vi "PickAndPlaceOnTape.vi"() -> ()   [LabVIEW 2021]
panel:
  in  "GoHome":bool
  in  "Operations":T1={"GoToToolPos"=TRUE, "PickTool"=TRUE, "GoToSenPCB"=TRUE, "PickSiPCB"=TRUE, "GoToBP"=TRUE, "DropTool"=TRUE}
  out "ZoneBasedFileNameStarting":string
  in  "Tape_PositionPartialFileName":string="Other_Position.txt"
  in  "PUT_PositionPartialFileName":string="PUT_Position.txt"
  in  "AssemblyPositionPartialFileName":string="Other_Position.txt"
  in  "BaseDirectory":string="C:\\Users\\TTUHEP\\Documents\\LabVIEW\\GantryPrograms\\Configs\\"
  out "Assembly_XYZU":dbl[](array[numeric])
  out "PUT_XYZU":dbl[](array[numeric])
  out "PUT rotation":dbl
  in  "FastZDrop":dbl=65.0
  in  "FastZToolPick":dbl=85.0
  in  "FastZSiPCBPick":dbl=65.0
  in  "LineNo":u8
  in  "ZSpeed":dbl=10.0
  in  "XYSpeed":dbl=100.0
  out "BPHBXYZU":dbl[](array[numeric])
  out "Error Out":errorcluster
  in  "Error In":errorcluster
  in  "VacuumStates":path=path "C:/Users/TTUHEP/Documents/LabVIEW/GantryPrograms/Configs/TapeCompPickPlaceVacuumStates.json"
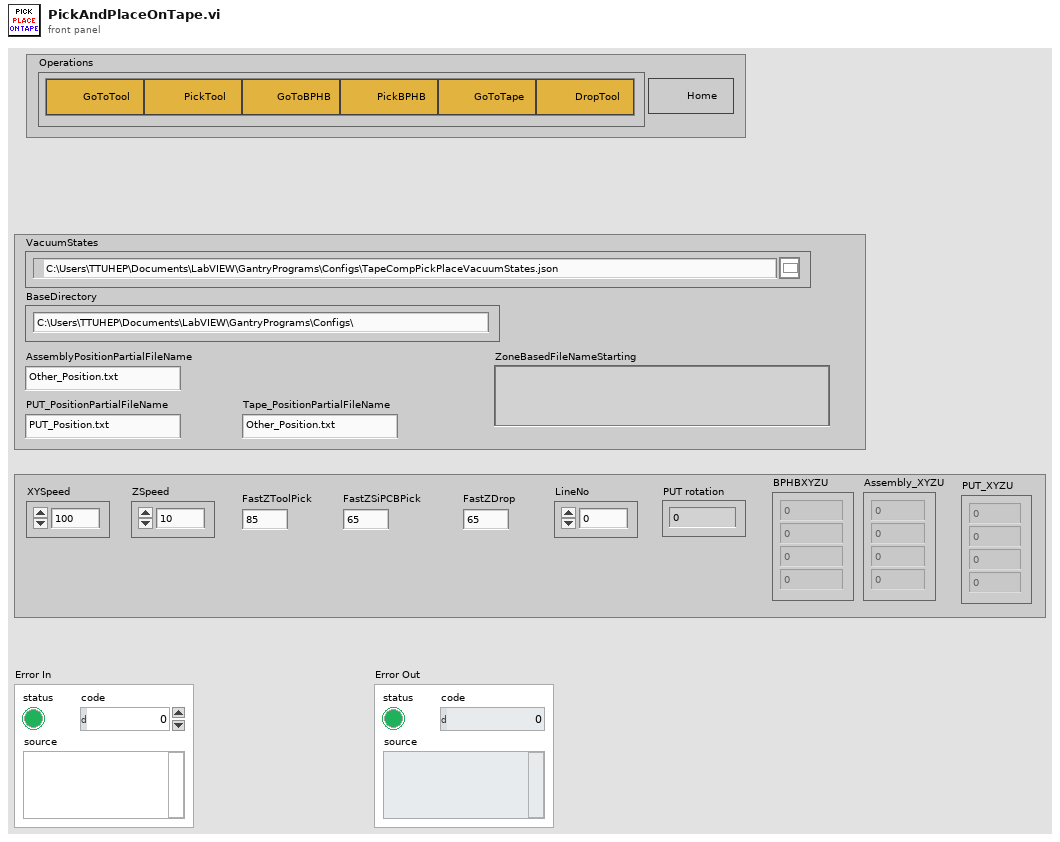
[diagram p1: front panel]
types:
  T1 = cluster{"GoToToolPos":bool, "PickTool":bool, "GoToSenPCB":bool, "PickSiPCB":bool, "GoToBP":bool, "DropTool":bool}
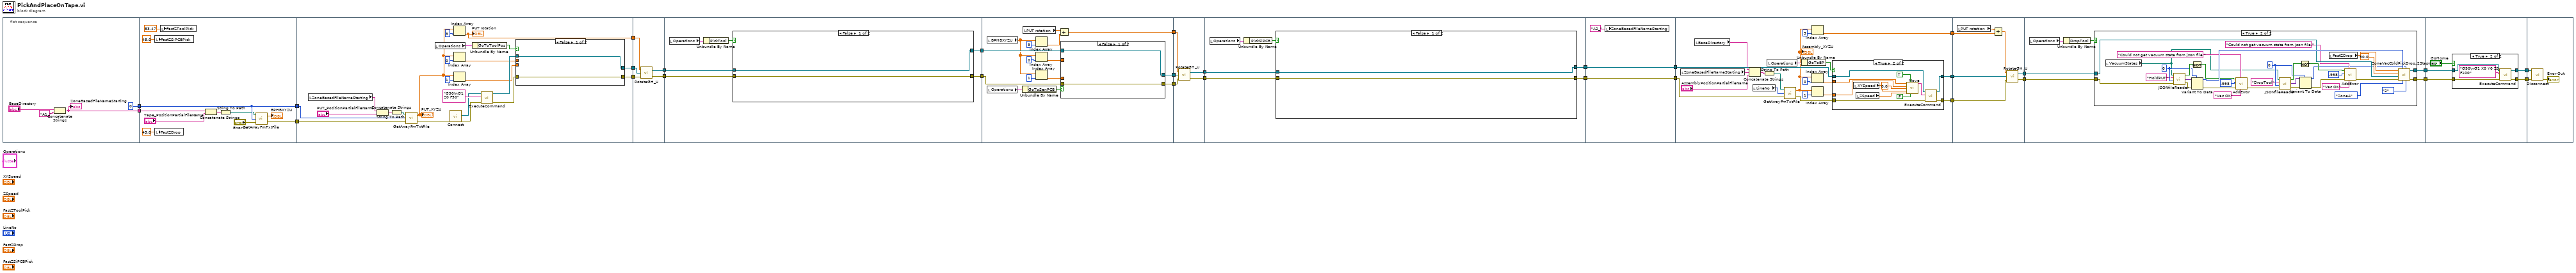
[diagram p0: block diagram]
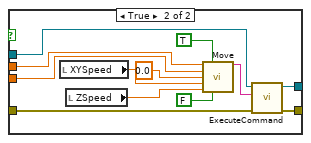
[diagram p2: hidden frame]
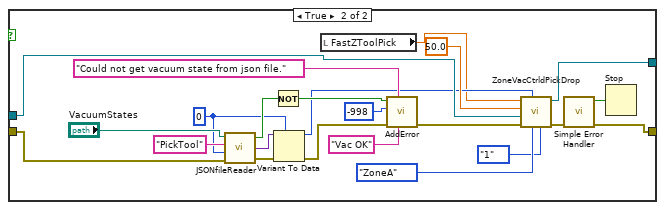
[diagram p3: hidden frame]
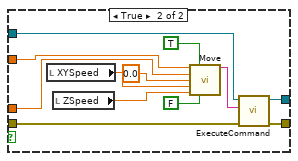
[diagram p4: hidden frame]
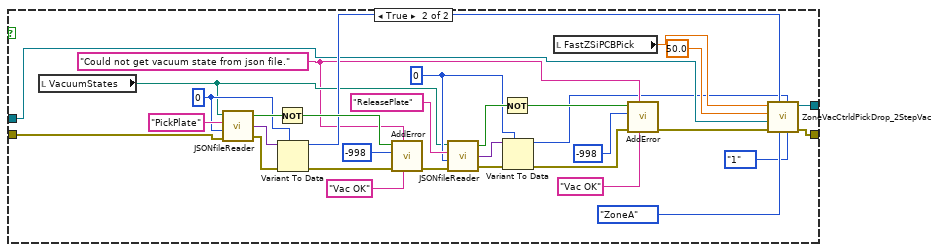
[diagram p5: hidden frame]
diagram:
  n1 = flat-sequence {
    tunnel: [u8 0 ("LineNo")] -> w11
    tunnel: [w31] -> w9
    tunnel: [w43] -> w12
    tunnel: w11 -> [w41]
    tunnel: [w41] -> w10
    tunnel: w9 -> [w40]
    tunnel: [w57] -> w29
    tunnel: [w56] -> w28
    tunnel: [w55] -> w27
    tunnel: w12 -> [w53]
    tunnel: w10 -> [w54]
    tunnel: w29 -> [w86]
    tunnel: w28 -> [w85]
    tunnel: w27 -> [w84]
    tunnel: [w83] -> w26
    tunnel: [w82] -> w25
    tunnel: w26 -> [w90]
    tunnel: w25 -> [w89]
    tunnel: [w88] -> w24
    tunnel: [w87] -> w23
    tunnel: w24 -> [w125]
    tunnel: w23 -> [w124]
    tunnel: [w118] -> w22
    tunnel: [w123] -> w21
    tunnel: [w122] -> w20
    tunnel: w22 -> [w151]
    tunnel: w21 -> [w150]
    tunnel: w20 -> [w149]
    tunnel: [w148] -> w19
    tunnel: [w147] -> w18
    tunnel: w19 -> [w155]
    tunnel: w18 -> [w154]
    tunnel: [w153] -> w8
    tunnel: [w152] -> w6
    tunnel: w8 -> [w194]
    tunnel: [w194] -> w7
    tunnel: w6 -> [w193]
    tunnel: [w193] -> w5
    tunnel: w7 -> [w206]
    tunnel: w5 -> [w205]
    tunnel: [w203] -> w17
    tunnel: [w202] -> w16
    tunnel: [w201] -> w15
    tunnel: w17 -> [w235]
    tunnel: w16 -> [w234]
    tunnel: w15 -> [w232]
    tunnel: [w230] -> w14
    tunnel: [w229] -> w13
    tunnel: w14 -> [w239]
    tunnel: w13 -> [w238]
    tunnel: [w237] -> w4
    tunnel: [w236] -> w2
    tunnel: w4 -> [w280]
    tunnel: [w277] -> w3
    tunnel: w2 -> [w279]
    tunnel: [w278] -> w1
    tunnel: w3 -> [w291]
    tunnel: w1 -> [w290]
    frame #0 {
      n2 = Concatenate Strings("BaseDirectory", "A1_") -> (w31:string)
      "ZoneBasedFileNameStarting" <- w31
    }
    frame #1 {
      n3 = local write "FastZSiPCBPick"(45.0 ("FastZSiPCBPick")) -> ()
      n4 = local write "FastZDrop"(45.0 ("FastZDrop")) -> ()
      n5 = local write "FastZToolPick"(83.47 ("FastZToolPick")) -> ()
      n6 = Concatenate Strings(w40, "Tape_PositionPartialFileName") -> (w36:string)
      n7 = String To Path(string=w36) -> (path=w35:path)
      n8 = call "GetArrayFmTxtFile.vi"("error in"="Error In", "LineNo."=w41, "TextFile"=w35) -> ("error out"=w43:errorcluster, "Array"=→"BPHBXYZU":dbl[])
    }
    frame #2 {
      n9 = local read "ZoneBasedFileNameStarting"() -> (w49:string)
      n10 = Concatenate Strings(w49, "PUT_PositionPartialFileName") -> (w48:string)
      n11 = String To Path(string=w48) -> (path=w47:path)
      n12 = call "GetArrayFmTxtFile.vi"("error in"=w53, "LineNo."=w54, "TextFile"=w47) -> ("error out"=w46:errorcluster, "Array"=w51:dbl[])
      "PUT_XYZU" <- w51
      n13 = local read "Operations"() -> (w64:T1)
      n14 = call "Connect.vi"("error in (no error)"=w46) -> ("error out"=w45:errorcluster, "controller"=w52:refnum<k24>)  [unwired: 9 in]
      n15 = Index Array(array=w51, index=3) -> (element=w55:dbl)
      "PUT rotation" <- w55
      n16 = Index Array(array=w51, index=0) -> (element=w59:dbl)
      n17 = Index Array(array=w51, index=1) -> (element=w58:dbl)
      n18 = Unbundle By Name(w64) -> ("GoToToolPos"=w63:bool)
      n19 = call "ExecuteCommand.vi"("error in (no error)"=w45, "Command Code"="G90\nG1 Z0 F50", "controller in"=w52) -> ("error out"=w67:errorcluster, "controller out"=w66:refnum<k24>)  [unwired: 6 in, 1 out]
      n20 = case shown="False" w63 {
        tunnel: w66 -> [w69 w78]
        tunnel: w67 -> [w68 w77]
        tunnel: [w68 w76] -> w57
        tunnel: [w69 w75] -> w56
        tunnel: w59 -> [_ w74]
        tunnel: w58 -> [_ w73]
        frame False {
        }
        frame True {
          n21 = local read "XYSpeed"() -> (w71:dbl)
          n22 = local read "ZSpeed"() -> (w70:dbl)
          n23 = call "Move.vi"("X"=w74, "Absolute"=TRUE, "Y"=w73, "Z"=0.0, "SpeedXY (mm/s)"=w71, "SpeedZ (mm/s)"=w70, "Move Z first"=FALSE) -> ("Position Gcode"=w79:string)  [unwired: 8 in]
          n24 = call "ExecuteCommand.vi"("error in (no error)"=w77, "Command Code"=w79, "controller in"=w78) -> ("error out"=w76:errorcluster, "controller out"=w75:refnum<k24>)  [unwired: 6 in, 1 out]
        }
      }
    }
    frame #3 {
      n25 = call "RotateGH_U.vi"("error in (no error)"=w86, "controller in"=w85, "U"=w84) -> ("error out"=w83:errorcluster, "controller out"=w82:refnum<k24>)
    }
    frame #4 {
      n26 = local read "Operations"() -> (w92:T1)
      n27 = Unbundle By Name(w92) -> ("PickTool"=w91:bool)
      n28 = case shown="False" w91 {
        tunnel: w90 -> [w94 w105]
        tunnel: w89 -> [w93 w116]
        tunnel: [w94 w97] -> w88
        tunnel: [w93 w101] -> w87
        frame False {
        }
        frame True {
          w108 = u8 0
          n29 = call "JSONfileReader.vi"("error in"=w105, "Variant"=w108, "ItemName"="PickTool", "FileIn"="VacuumStates") -> ("error out"=w103:errorcluster, "Data"=w107:variant, "Found"=w112:bool)
          n30 = Not(x=w112) -> (.not. x?=w113:bool)
          n31 = Variant To Data(error in=w103, type=w108, Variant=w107) -> (data=w106:u8, error out=w102:errorcluster)
          n32 = local read "FastZToolPick"() -> (w100:dbl)
          n33 = call "AddError.vi"("NoErrorMessage"="Vac OK", "ErrorMessage"="Could not get vacuum state from json file.", "error in"=w102, "code"=-998, "Error?"=w113) -> ("Error out"=w104:errorcluster)  [unwired: 6 in]
          n34 = call "ZoneVacCtrldPickDrop.vi"("Position"=enum16{"1", "2"}."1", "Zone"=enum16{"ZoneA", "ZoneB", "ZoneC", "ZoneD"}."ZoneA", "VacuumState"=w106, "error in (no error)"=w104, "controller in"=w116, "Zspeed"=50.0, "Z"=w100) -> ("error out"=w98:errorcluster, "controller out"=w101:refnum<k24>)  [unwired: 3 in]
          n35 = call <vilib>:"Simple Error Handler.vi"("error in (no error)"=w98) -> ("error?"=w99:bool, "error out"=w97:errorcluster)  [unwired: 4 in, 3 out]
          n36 = Stop(stop? (T)=w99) -> ()
        }
      }
    }
    frame #5 {
      n37 = local read "BPHBXYZU"() -> (w121:dbl[])
      n38 = local read "Operations"() -> (w129:T1)
      n39 = Unbundle By Name(w129) -> ("GoToSenPCB"=w130:bool)
      n40 = local read "PUT rotation"() -> (w120:dbl)
      n41 = Index Array(array=w121, index=3) -> (element=w119:dbl)
      n42 = Index Array(array=w121, index=0) -> (element=w131:dbl)
      n43 = Index Array(array=w121, index=1) -> (element=w132:dbl)
      n44 = Add(x=w120, y=w119) -> (x+y=w118:dbl)
      n45 = case shown="False" w130 {
        tunnel: w124 -> [w134 w143]
        tunnel: w125 -> [w133 w142]
        tunnel: [w133 w141] -> w122
        tunnel: [w134 w140] -> w123
        tunnel: w131 -> [_ w139]
        tunnel: w132 -> [_ w138]
        frame False {
        }
        frame True {
          n46 = local read "XYSpeed"() -> (w135:dbl)
          n47 = local read "ZSpeed"() -> (w136:dbl)
          n48 = call "Move.vi"("X"=w139, "Absolute"=TRUE, "Y"=w138, "Z"=0.0, "SpeedXY (mm/s)"=w135, "SpeedZ (mm/s)"=w136, "Move Z first"=FALSE) -> ("Position Gcode"=w144:string)  [unwired: 8 in]
          n49 = call "ExecuteCommand.vi"("error in (no error)"=w142, "Command Code"=w144, "controller in"=w143) -> ("error out"=w141:errorcluster, "controller out"=w140:refnum<k24>)  [unwired: 6 in, 1 out]
        }
      }
    }
    frame #6 {
      n50 = call "RotateGH_U.vi"("error in (no error)"=w149, "controller in"=w150, "U"=w151) -> ("error out"=w147:errorcluster, "controller out"=w148:refnum<k24>)
    }
    frame #7 {
      n51 = local read "Operations"() -> (w156:T1)
      n52 = Unbundle By Name(w156) -> ("PickSiPCB"=w157:bool)
      n53 = case shown="False" w157 {
        tunnel: w154 -> [w159 w182]
        tunnel: w155 -> [w158 w176]
        tunnel: [w159 w179] -> w152
        tunnel: [w158 w178] -> w153
        frame False {
        }
        frame True {
          w170 = u8 0
          w185 = u8 0
          w163 = "Could not get vacuum state from json file." ("ErrorMessage")
          n54 = local read "VacuumStates"() -> (w166:path)
          n55 = call "JSONfileReader.vi"("error in"=w182, "Variant"=w185, "ItemName"="PickPlate", "FileIn"=w166) -> ("error out"=w181:errorcluster, "Data"=w184:variant, "Found"=w188:bool)
          n56 = Not(x=w188) -> (.not. x?=w189:bool)
          n57 = Variant To Data(error in=w181, type=w185, Variant=w184) -> (data=w183:u8, error out=w180:errorcluster)
          n58 = call "AddError.vi"("NoErrorMessage"="Vac OK", "ErrorMessage"=w163, "error in"=w180, "code"=-998, "Error?"=w189) -> ("Error out"=w165:errorcluster)  [unwired: 6 in]
          n59 = call "JSONfileReader.vi"("error in"=w165, "Variant"=w170, "ItemName"="ReleasePlate", "FileIn"=w166) -> ("error out"=w168:errorcluster, "Data"=w169:variant, "Found"=w173:bool)
          n60 = Not(x=w173) -> (.not. x?=w174:bool)
          n61 = Variant To Data(error in=w168, type=w170, Variant=w169) -> (data=w162:u8, error out=w167:errorcluster)
          n62 = local read "FastZSiPCBPick"() -> (w177:dbl)
          n63 = call "AddError.vi"("NoErrorMessage"="Vac OK", "ErrorMessage"=w163, "error in"=w167, "code"=-998, "Error?"=w174) -> ("Error out"=w164:errorcluster)  [unwired: 6 in]
          n64 = call "ZoneVacCtrldPickDrop_2StepVac.vi"("Position"=enum16{"1", "2"}."1", "VacuumState2"=w162, "Zone"=enum16{"ZoneA", "ZoneB", "ZoneC", "ZoneD"}."ZoneA", "VacuumState1"=w183, "error in (no error)"=w164, "controller in"=w176, "Zspeed"=50.0, "Z"=w177) -> ("error out"=w179:errorcluster, "controller out"=w178:refnum<k24>)  [unwired: 2 in]
        }
      }
    }
    frame #8 {
      n65 = local write "ZoneBasedFileNameStarting"("A2_") -> ()
    }
    frame #9 {
      n66 = local read "ZoneBasedFileNameStarting"() -> (w199:string)
      n67 = local read "BaseDirectory"() -> (w195:string)
      n68 = Concatenate Strings(w195, w199, "AssemblyPositionPartialFileName") -> (w197:string)
      n69 = local read "LineNo"() -> (w207:u8)
      n70 = String To Path(string=w197) -> (path=w196:path)
      n71 = local read "Operations"() -> (w214:T1)
      n72 = call "GetArrayFmTxtFile.vi"("error in"=w205, "LineNo."=w207, "TextFile"=w196) -> ("error out"=w204:errorcluster, "Array"=w200:dbl[])
      "Assembly_XYZU" <- w200
      n73 = Unbundle By Name(w214) -> ("GoToBP"=w213:bool)
      n74 = Index Array(array=w200, index=3) -> (element=w201:dbl)
      n75 = Index Array(array=w200, index=0) -> (element=w212:dbl)
      n76 = Index Array(array=w200, index=1) -> (element=w211:dbl)
      n77 = case shown="True" w213 {
        tunnel: w206 -> [w216 w225]
        tunnel: w204 -> [w215 w224]
        tunnel: [w215 w223] -> w203
        tunnel: [w216 w222] -> w202
        tunnel: w212 -> [_ w221]
        tunnel: w211 -> [_ w220]
        frame False {
        }
        frame True {
          n78 = local read "XYSpeed"() -> (w217:dbl)
          n79 = local read "ZSpeed"() -> (w218:dbl)
          n80 = call "Move.vi"("X"=w221, "Absolute"=TRUE, "Y"=w220, "Z"=0.0, "SpeedXY (mm/s)"=w217, "SpeedZ (mm/s)"=w218, "Move Z first"=FALSE) -> ("Position Gcode"=w226:string)  [unwired: 8 in]
          n81 = call "ExecuteCommand.vi"("error in (no error)"=w224, "Command Code"=w226, "controller in"=w225) -> ("error out"=w223:errorcluster, "controller out"=w222:refnum<k24>)  [unwired: 6 in, 1 out]
        }
      }
    }
    frame #10 {
      n82 = local read "PUT rotation"() -> (w233:dbl)
      n83 = Add(x=w233, y=w232) -> (x+y=w231:dbl)
      n84 = call "RotateGH_U.vi"("error in (no error)"=w235, "controller in"=w234, "U"=w231) -> ("error out"=w230:errorcluster, "controller out"=w229:refnum<k24>)
    }
    frame #11 {
      n85 = local read "Operations"() -> (w241:T1)
      n86 = Unbundle By Name(w241) -> ("DropTool"=w240:bool)
      n87 = case shown="True" w240 {
        tunnel: w239 -> [w243 w263]
        tunnel: w238 -> [w242 w262]
        tunnel: [w243 w261] -> w237
        tunnel: [w242 w260] -> w236
        frame False {
        }
        frame True {
          w254 = u8 0
          w269 = u8 0
          n88 = local read "VacuumStates"() -> (w249:path)
          n89 = call "JSONfileReader.vi"("error in"=w263, "Variant"=w269, "ItemName"="HoldPUT", "FileIn"=w249) -> ("error out"=w274:errorcluster, "Data"=w272:variant, "Found"=w271:bool)
          n90 = Not(x=w271) -> (.not. x?=w270:bool)
          n91 = Variant To Data(error in=w274, type=w269, Variant=w272) -> (data=w273:u8, error out=w275:errorcluster)
          n92 = call "AddError.vi"("NoErrorMessage"="Vac OK", "ErrorMessage"="Could not get vacuum state from json file.", "error in"=w275, "code"=-998, "Error?"=w270) -> ("Error out"=w248:errorcluster)  [unwired: 6 in]
          n93 = call "JSONfileReader.vi"("error in"=w248, "Variant"=w254, "ItemName"="DropTool", "FileIn"=w249) -> ("error out"=w258:errorcluster, "Data"=w257:variant, "Found"=w256:bool)
          n94 = Not(x=w256) -> (.not. x?=w255:bool)
          n95 = Variant To Data(error in=w258, type=w254, Variant=w257) -> (data=w246:u8, error out=w259:errorcluster)
          n96 = local read "FastZDrop"() -> (w276:dbl)
          n97 = call "AddError.vi"("NoErrorMessage"="Vac OK", "ErrorMessage"="Could not get vacuum state from json file.", "error in"=w259, "code"=-998, "Error?"=w255) -> ("Error out"=w247:errorcluster)  [unwired: 6 in]
          n98 = call "ZoneVacCtrldPickDrop_2StepVac.vi"("Position"=enum16{"1", "2"}."2", "VacuumState2"=w246, "Zone"=enum16{"ZoneA", "ZoneB", "ZoneC", "ZoneD"}."ZoneA", "VacuumState1"=w273, "error in (no error)"=w247, "controller in"=w262, "Zspeed"=50.0, "Z"=w276) -> ("error out"=w261:errorcluster, "controller out"=w260:refnum<k24>)  [unwired: 2 in]
        }
      }
    }
    frame #12 {
      n99 = case shown="True" "GoHome" {
        tunnel: [w283 w284] -> w277
        tunnel: w280 -> [w283 w287]
        tunnel: w279 -> [w282 w286]
        tunnel: [w282 w285] -> w278
        frame False {
        }
        frame True {
          n100 = call "ExecuteCommand.vi"("error in (no error)"=w287, "Command Code"="G90\nG1 X0 Y0 Z0 F100", "controller in"=w286) -> ("error out"=w284:errorcluster, "controller out"=w285:refnum<k24>)  [unwired: 6 in, 1 out]
        }
      }
    }
    frame #13 {
      n101 = call "Disconnect.vi"("error in (no error)"=w291, "controller"=w290) -> ("error out"=→"Error Out":errorcluster)  [unwired: 9 in]
    }
  }
